vi "ReadDet_G.vi"(8 "error in (no error)":errorcluster, 9 "data":variant, 11 "Control-Client in":refnum<class "Control-Client.lvclass">) -> (0 "error out":errorcluster, 3 "Control-Client out":refnum<class "Control-Client.lvclass">)   [LabVIEW 2019, in "Control-Client.lvclass"]
uses:
  Control-Client.lvclass
  dependecies/ControlsVIs/Clusters-def/Det-Reply-to-Read.ctl
  dependecies/ControlsVIs/Clusters-def/Def_signals_from_DET.ctl
  dependecies/ControlsVIs/Clusters-def/SERVER-Commands.ctl
  dependecies/ControlsVIs/Clusters-def/Message types.ctl
  dependecies/ControlsVIs/Clusters-def/Def_Vis_Addrow.ctl
  Experiments/Experiment.lvclass/Experiment.ctl
  Control-Client.lvclass/Control-Client.ctl
  Experiments/Experiment.lvclass
  Control-Server/Control-Server.lvclass
  Detector/Detector.lvclass
panel:
  in  "?":T1
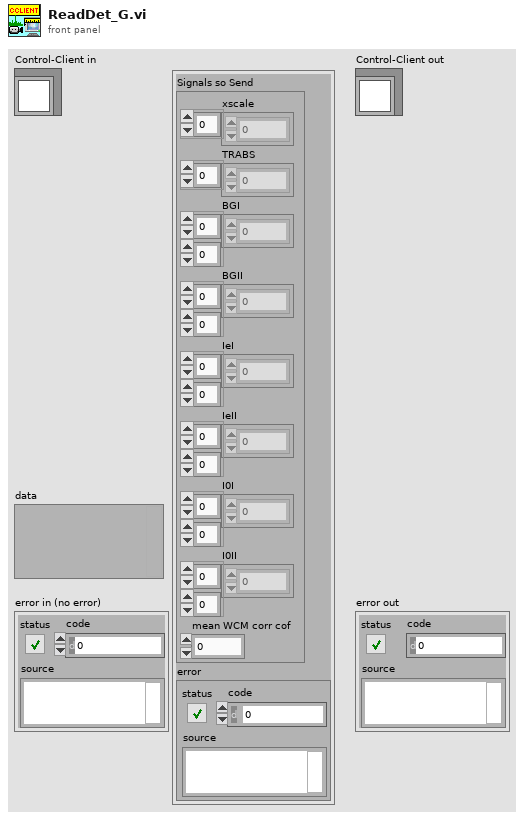
[diagram p1: front panel]
types:
  T1 = typedef "Detector.lvclass/Det-Reply-to-Read.ctl" = cluster{"Signals so Send":T2, "error":errorcluster}
  T2 = typedef "Detector.lvclass/Def_signals_from_DET.ctl" = cluster{"xscale":sgl[], "TRABS":sgl[], "BGI":sgl[][], "BGII":sgl[][], "IeI":sgl[][], "IeII":sgl[][], "I0I":sgl[][], "I0II":sgl[][], "mean WCM corr cof":dbl}
  T3 = typedef "Control-Client.lvclass/Def_Vis_Addrow.ctl" = cluster{"row":sgl[], "timedelays":dbl[]}
  T4 = typedef "Message types.ctl" = string
  T5 = typedef "Control-Server.lvclass/SERVER-Commands.ctl" = string
  T6 = typedef "Control-Client.lvclass/Delays-refs_CLIENT.ctl" = cluster{"# points":refnum<vi>, "Step, ps":refnum<vi>, "OZ, ps":refnum<vi>, "# current":refnum<vi>, "RDT, ps":refnum<vi>, "Total length, ps":refnum<vi>, "Kinetics length, ps":refnum<vi>, "Real zero, ps":refnum<vi>, "# par point":refnum<vi>}
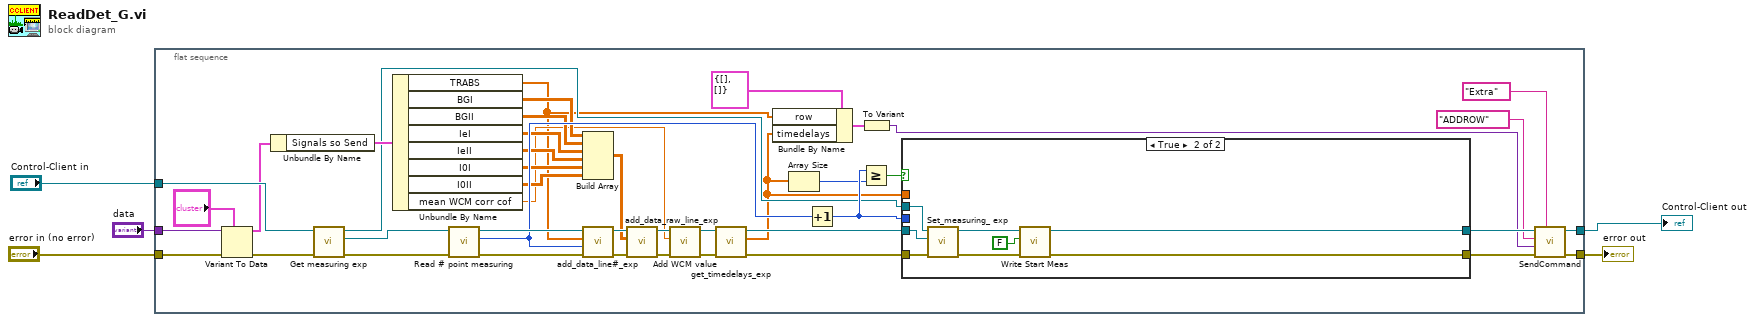
[diagram p0: block diagram]
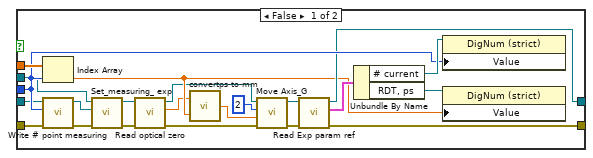
[diagram p2: hidden frame]
diagram:
  n1 = flat-sequence {
    tunnel: "Control-Client in" -> [w45]
    tunnel: "error in (no error)" -> [w43]
    tunnel: "data" -> [w42]
    tunnel: [w15] -> w2
    tunnel: [w14] -> w1
    frame #0 {
      n2 = Variant To Data(error in=w43, type="?", Variant=w42) -> (data=w44:T1, error out=w46:errorcluster)
      n3 = Unbundle By Name(w44) -> ("Signals so Send"=w32:T2)
      n4 = call "Get measuring exp.vi"("error in (no error)"=w46, "Control-Client in"=w45) -> ("error out"=w47:errorcluster, "Measured experiment"=w48:refnum<class "Experiment.lvclass">, "Control-Client out"=w17:refnum<class "Control-Client.lvclass">)  [unwired: 7 in]
      n5 = Unbundle By Name(w32) -> ("TRABS"=w8:sgl[], "BGI"=w31:sgl[][], "BGII"=w30:sgl[][], "IeI"=w29:sgl[][], "IeII"=w28:sgl[][], "I0I"=w27:sgl[][], "I0II"=w26:sgl[][], "mean WCM corr cof"=w21:dbl)
      n6 = call "Read # point measuring.vi"("error in (no error)"=w47, "Experiment in"=w48) -> ("error out"=w36:errorcluster, "# point measuring"=w33:i32, "Experiment out"=w37:refnum<class "Experiment.lvclass">)  [unwired: 7 in]
      n7 = Build Array(w31, w30, w29, w28, w27, w26) -> (w20:sgl[][][])
      n8 = call "add_data_line#_exp.vi"("error in (no error)"=w36, "#"=w33, "add Array"=w8, "Experiment.lvclass in"=w37) -> ("error out"=w34:errorcluster, "Experiment.lvclass out"=w35:refnum<class "Experiment.lvclass">)  [unwired: 6 in]
      n9 = call "add_data_raw_line_exp.vi"("error in (no error)"=w34, "add Data"=w20, "Experiment.lvclass in"=w35) -> ("error out"=w22:errorcluster, "Experiment.lvclass out"=w25:refnum<class "Experiment.lvclass">)  [unwired: 7 in]
      n10 = call-dynamic "Add WCM value.vi"("error in (no error)"=w22, "WCM value"=w21, "Experiment in"=w25) -> ("error out"=w23:errorcluster, "Experiment out"=w24:refnum<class "Experiment.lvclass">)  [unwired: 7 in]
      n11 = call "get_timedelays_exp.vi"("error in (no error)"=w23, "Experiment.lvclass in"=w24) -> ("error out"=w18:errorcluster, "timedelays"=w6:dbl[], "Experiment.lvclass out"=w19:refnum<class "Experiment.lvclass">)  [unwired: 7 in]
      n12 = Bundle By Name(cluster=T3 {"row"=[], "timedelays"=[]} ("Cluster"), "row"=w8, "timedelays"=w6) -> (w9:T3)
      n13 = Array Size(array=w6) -> (size(s)=w39:i32)
      n14 = Increment(x=w33) -> (x+1=w40:i32)
      n15 = Greater Or Equal?(x=w40, y=w39) -> (x >= y?=w38:bool)
      n16 = To Variant(anything=w9) -> (Variant=w7:variant)
      n17 = case shown="True" w38 {
        tunnel: w6 -> [w70 _]
        tunnel: w40 -> [w63 _]
        tunnel: [w59 w74] -> w13
        tunnel: w18 -> [w67 w76]
        tunnel: [w58 w73] -> w16
        tunnel: w17 -> [w54 w72]
        tunnel: w19 -> [w55 w71]
        frame False {
          n18 = Index Array(array=w70, index=w63) -> (element=w56:dbl)
          n19 = call "Write # point measuring.vi"("error in (no error)"=w67, "# point measuring"=w63, "Experiment in"=w55) -> ("error out"=w65:errorcluster, "Experiment out"=w66:refnum<class "Experiment.lvclass">)  [unwired: 7 in]
          n20 = call "Set_measuring_ exp.vi"("error in (no error)"=w65, "Experiment"=w66, "Control-Client in"=w54) -> ("error out"=w52:errorcluster, "Control-Client out"=w53:refnum<class "Control-Client.lvclass">)  [unwired: 7 in]
          n21 = call-dynamic "Read optical zero.vi"("error in (no error)"=w52, "Control-Client in"=w53) -> ("error out"=w51:errorcluster, "optical zero"=w49:dbl, "Control-Client out"=w50:refnum<class "Control-Client.lvclass">)  [unwired: 7 in]
          n22 = call "convertps-to-mm.vi"("ps"=w56, "Real zero"=w49) -> ("mm"=w69:dbl)
          n23 = call "Move Axis_G.vi"("error in (no error)"=w51, "Where, mm"=w69, "Axis"=2, "Control-Client in"=w50) -> ("error out"=w62:errorcluster, "Control-Client out"=w61:refnum<class "Control-Client.lvclass">)  [unwired: 6 in]
          n24 = call "Read Exp param ref.vi"("error in (no error)"=w62, "Control-Client in"=w61) -> ("error out"=w58:errorcluster, "Exp param ref"=w60:T6, "Control-Client out"=w59:refnum<class "Control-Client.lvclass">)  [unwired: 7 in]
          n25 = Unbundle By Name(w60) -> ("# current"=w64:refnum<vi>, "RDT, ps"=w57:refnum<vi>)
          n26 = property class="DigNum (strict)"(reference=w64, "Value"=w63) -> ()  [unwired: 1 in, 2 out]
          n27 = property class="DigNum (strict)"(reference=w57, "Value"=w56) -> ()  [unwired: 1 in, 2 out]
        }
        frame True {
          n28 = call "Set_measuring_ exp.vi"("error in (no error)"=w76, "Experiment"=w71, "Control-Client in"=w72) -> ("error out"=w75:errorcluster, "Control-Client out"=w77:refnum<class "Control-Client.lvclass">)  [unwired: 7 in]
          n29 = call "Write Start Meas.vi"("error in (no error)"=w75, "Start Meas"=FALSE, "Control-Client in"=w77) -> ("error out"=w73:errorcluster, "Control-Client out"=w74:refnum<class "Control-Client.lvclass">)  [unwired: 7 in]
        }
      }
      n30 = call "SendCommand.vi"("Message type"=T4 "Extra", "error in (no error)"=w16, "data"=w7, "Command"=T5 "ADDROW" ("Commands"), "Control-Client in"=w13) -> ("error out"=w15:errorcluster, "Control-Client out"=w14:refnum<class "Control-Client.lvclass">)  [unwired: 5 in]
    }
  }
  "error out" <- w2
  "Control-Client out" <- w1
